vi "Initialize Match Template.vi"(11 "base path":path=path "Fiducial_3_Dots.bmp") -> (3 "Pattern Matched Image":T1(plugin-control))   [LabVIEW 2019]
uses:
  <vilib>/vision/NI_Vision_Development_Module.lvlib
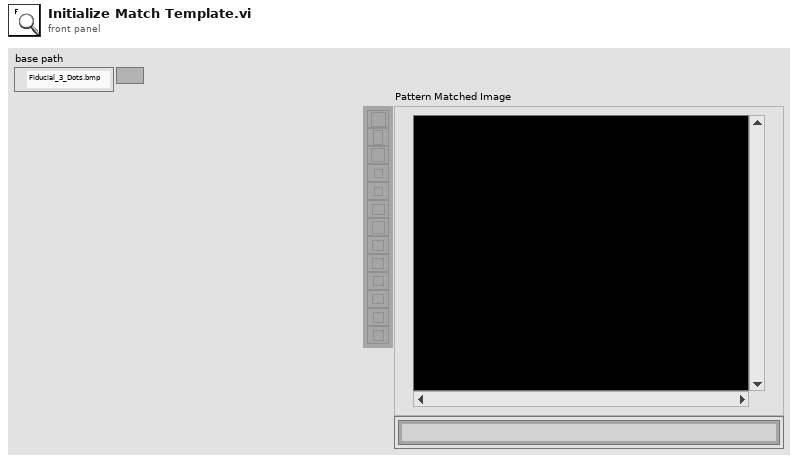
[diagram p1: front panel]
types:
  T1 = typedef "IMAQ Image.ctl" = refnum<image>
  T2 = typedef "Image Type" = u32
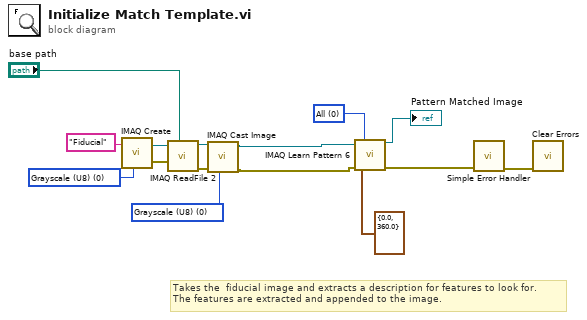
[diagram p0: block diagram]
diagram:
  w4 = T2 0 items=["Grayscale (U8)", "Grayscale (I16)", "Grayscale (SGL)", "Complex (CSG)", "RGB (U32)", "HSL (U32)", "RGB (U64)", "Grayscale (U16)"] ("Image Type")
  w8 = T2 0 items=["Grayscale (U8)", "Grayscale (I16)", "Grayscale (SGL)", "Complex (CSG)", "RGB (U32)", "HSL (U32)", "RGB (U64)", "Grayscale (U16)"] ("Image Type")
  w12 = 0 items=["All", "Low Discrepancy Sampling", "Grayscale Value Pyramid", "Gradients Pyramid"] ("Algorithm")
  # "Takes the  fiducial image and extracts a description for features to look for.\nThe features are extracted and appended to the image."
  n1 = call "IMAQ Create"("Image Name"="Fiducial", "Image Type"=w8) -> ("New Image"=w7:T1, "error out"=w10:errorcluster)  [unwired: 3 in]
  n2 = call "IMAQ ReadFile 2"("File Path"="base path", "error in (no error)"=w10, "Image"=w7) -> ("error out"=w6:errorcluster, "Image Out"=w5:T1)  [unwired: 4 in, 3 out]
  n3 = call "IMAQ Cast Image"("Image Type"=w4, "error in (no error)"=w6, "Image Src"=w5) -> ("error out"=w3:errorcluster, "Image Dst Out"=w2:T1)  [unwired: 7 in]
  n4 = call "IMAQ Learn Pattern 6"("Image"=w2, "Algorithm"=w12, "Angle Range"=cluster{"Start Angle":sgl, "End Angle":sgl} {"Start Angle"=0.0, "End Angle"=360.0}, "error in (no error)"=w3) -> ("Template Image Out"=→"Pattern Matched Image":T1, "error out"=w14:errorcluster)  [unwired: 9 in, 1 out]
  n5 = call <vilib>:"Simple Error Handler.vi"("error in (no error)"=w14) -> ("error out"=w15:errorcluster)  [unwired: 4 in, 4 out]
  n6 = call <vilib>:"Clear Errors.vi"("error in (no error)"=w15) -> ()  [unwired: 5 in, 2 out]
